vi "File_SortByDepth.vi"(1 "Paths":path[](array[path]), 3 "Ascending?":bool) -> (15 "Paths sorted":path[](array[path]))   [LabVIEW 2014]
doc: "Sorts path by depth"
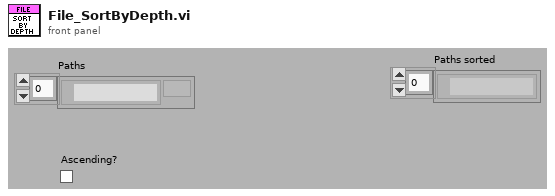
[diagram p1: front panel]
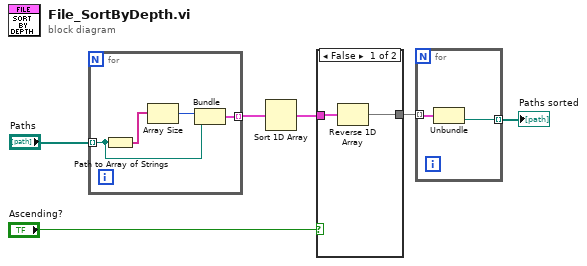
[diagram p0: block diagram]
diagram:
  n1 = for {
    tunnel: "Paths" -> [w8] mode=indexing
    tunnel: [w7] -> w5 mode=indexing
    n2 = Path to Array of Strings(0:w8) -> (2:w10:string[])  [unwired: 1 out]
    n3 = Array Size(array=w10) -> (size(s)=w9:i32)
    n4 = Bundle(w9, "Path"=w8) -> (w7:cluster{i32, "Path":path})  [unwired: 1 out]
  }
  n5 = Sort 1D Array(array=w5) -> (sorted array=w3:cluster{i32, "Path":path}[])
  n6 = case shown="False" "Ascending?" {
    tunnel: w3 -> [w12 w13]
    tunnel: [w11 w13] -> w2
    frame False {
      n7 = Reverse 1D Array(array=w12) -> (reversed array=w11:cluster{i32, "Path":path}[])
    }
    frame True {
    }
  }
  n8 = for {
    tunnel: w2 -> [w15] mode=indexing
    tunnel: [w14] -> w1 mode=indexing
    n9 = Unbundle(w15) -> ("Path"=w14:path)  [unwired: 1 out]
  }
  "Paths sorted" <- w1
